vi "柱塞泵调试界面.vi"() -> ()   [LabVIEW 2016, in "质控单元.lvlib"]
uses:
  <vilib>/Utility/miscctls.llb/LVPointTypeDef.ctl
  <vilib>/Analysis/6fits.llb/Curve Fitting Criteria.ctl
  <vilib>/Utility/config.llb/Write Key (U32).vi
  <vilib>/Analysis/NI_AALPro.lvlib
  <vilib>/Utility/config.llb/NI_LVConfig.lvlib
panel:
  out "关闭 2":bool=TRUE
  in  "枚举":enum16{"柱塞泵1", "柱塞泵2", "柱塞泵3", "柱塞泵4"}(ring)
  in  "柱塞泵4":bool
  in  "柱塞泵3":bool
  in  "柱塞泵2":bool
  in  "柱塞泵1":bool
  in  "注出体积选择":u16(ring) items=["0.1mL", "0.3mL", "0.5mL", "0.8mL", "1.0mL"]
  out "线性值":T1
  in  "读取":bool
  in  "写入":bool
  in  "柱塞泵枚举":enum16{"柱塞泵1", "柱塞泵2", "柱塞泵3", "柱塞泵4"}(ring)
  in  "启用计算":bool
  in  "标准体积 2":dbl
  in  "标准体积 3":dbl
  in  "实际体积 1":dbl
  in  "实际体积 2":dbl
  in  "实际体积 3":dbl
  in  "标准体积 4":dbl
  in  "实际体积 4":dbl
  in  "标准体积 5":dbl
  in  "实际体积 5":dbl
  in  "标准体积 1":dbl
  out "拟合方程":string
  out "r^2":dbl format="%_6g"
  in  "B 4":dbl caption="B4"
  in  "K 4":dbl caption="K4"
  in  "B 3":dbl caption="B3"
  in  "K 3":dbl caption="K3"
  in  "B 2":dbl caption="B2"
  in  "K 2":dbl caption="K2"
  in  "B":dbl caption="B1"
  in  "K":dbl caption="K1"
  in  "关闭":bool
  # "柱塞泵手动调试计算界面"
  # "柱塞泵启动控制"
  # "柱塞泵5点线性计算"
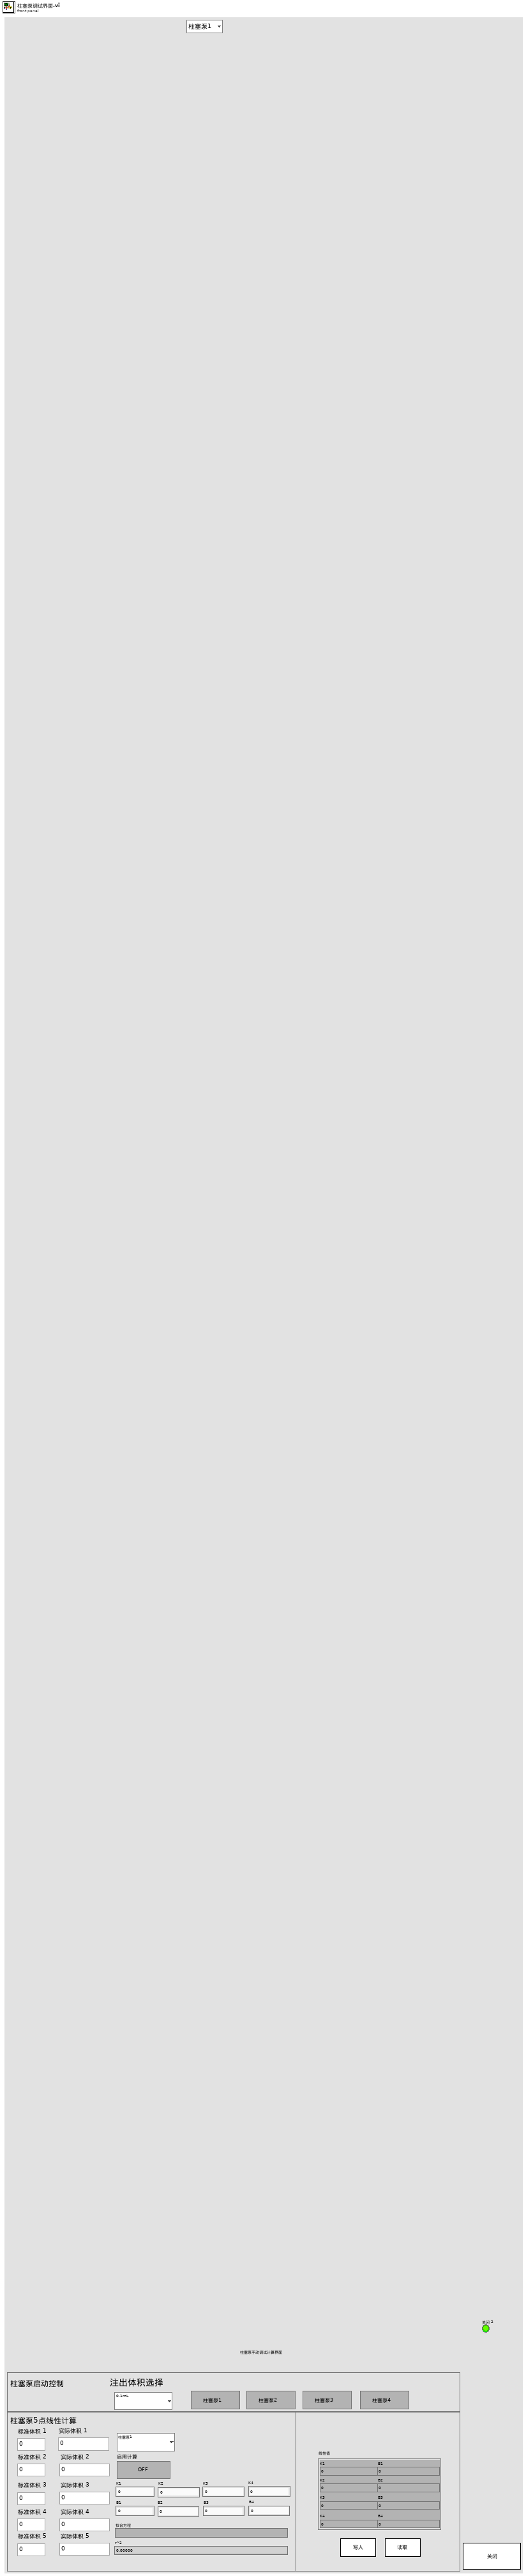
[diagram p1: front panel]
types:
  T1 = cluster{"K1":sgl, "B1":sgl, "K2":sgl, "B2":sgl, "K3":sgl, "B3":sgl, "K4":sgl, "B4":sgl}
  T2 = typedef "LVPointTypeDef.ctl" = cluster{"Horizontal":i16, "Vertical":i16}
  T3 = typedef "NI_LVConfig.lvlib/Config Data RefNum.ctl" = refnum<k1>
  T4 = typedef "NI_AALPro.lvlib/Curve Fitting Criteria.ctl" = u16
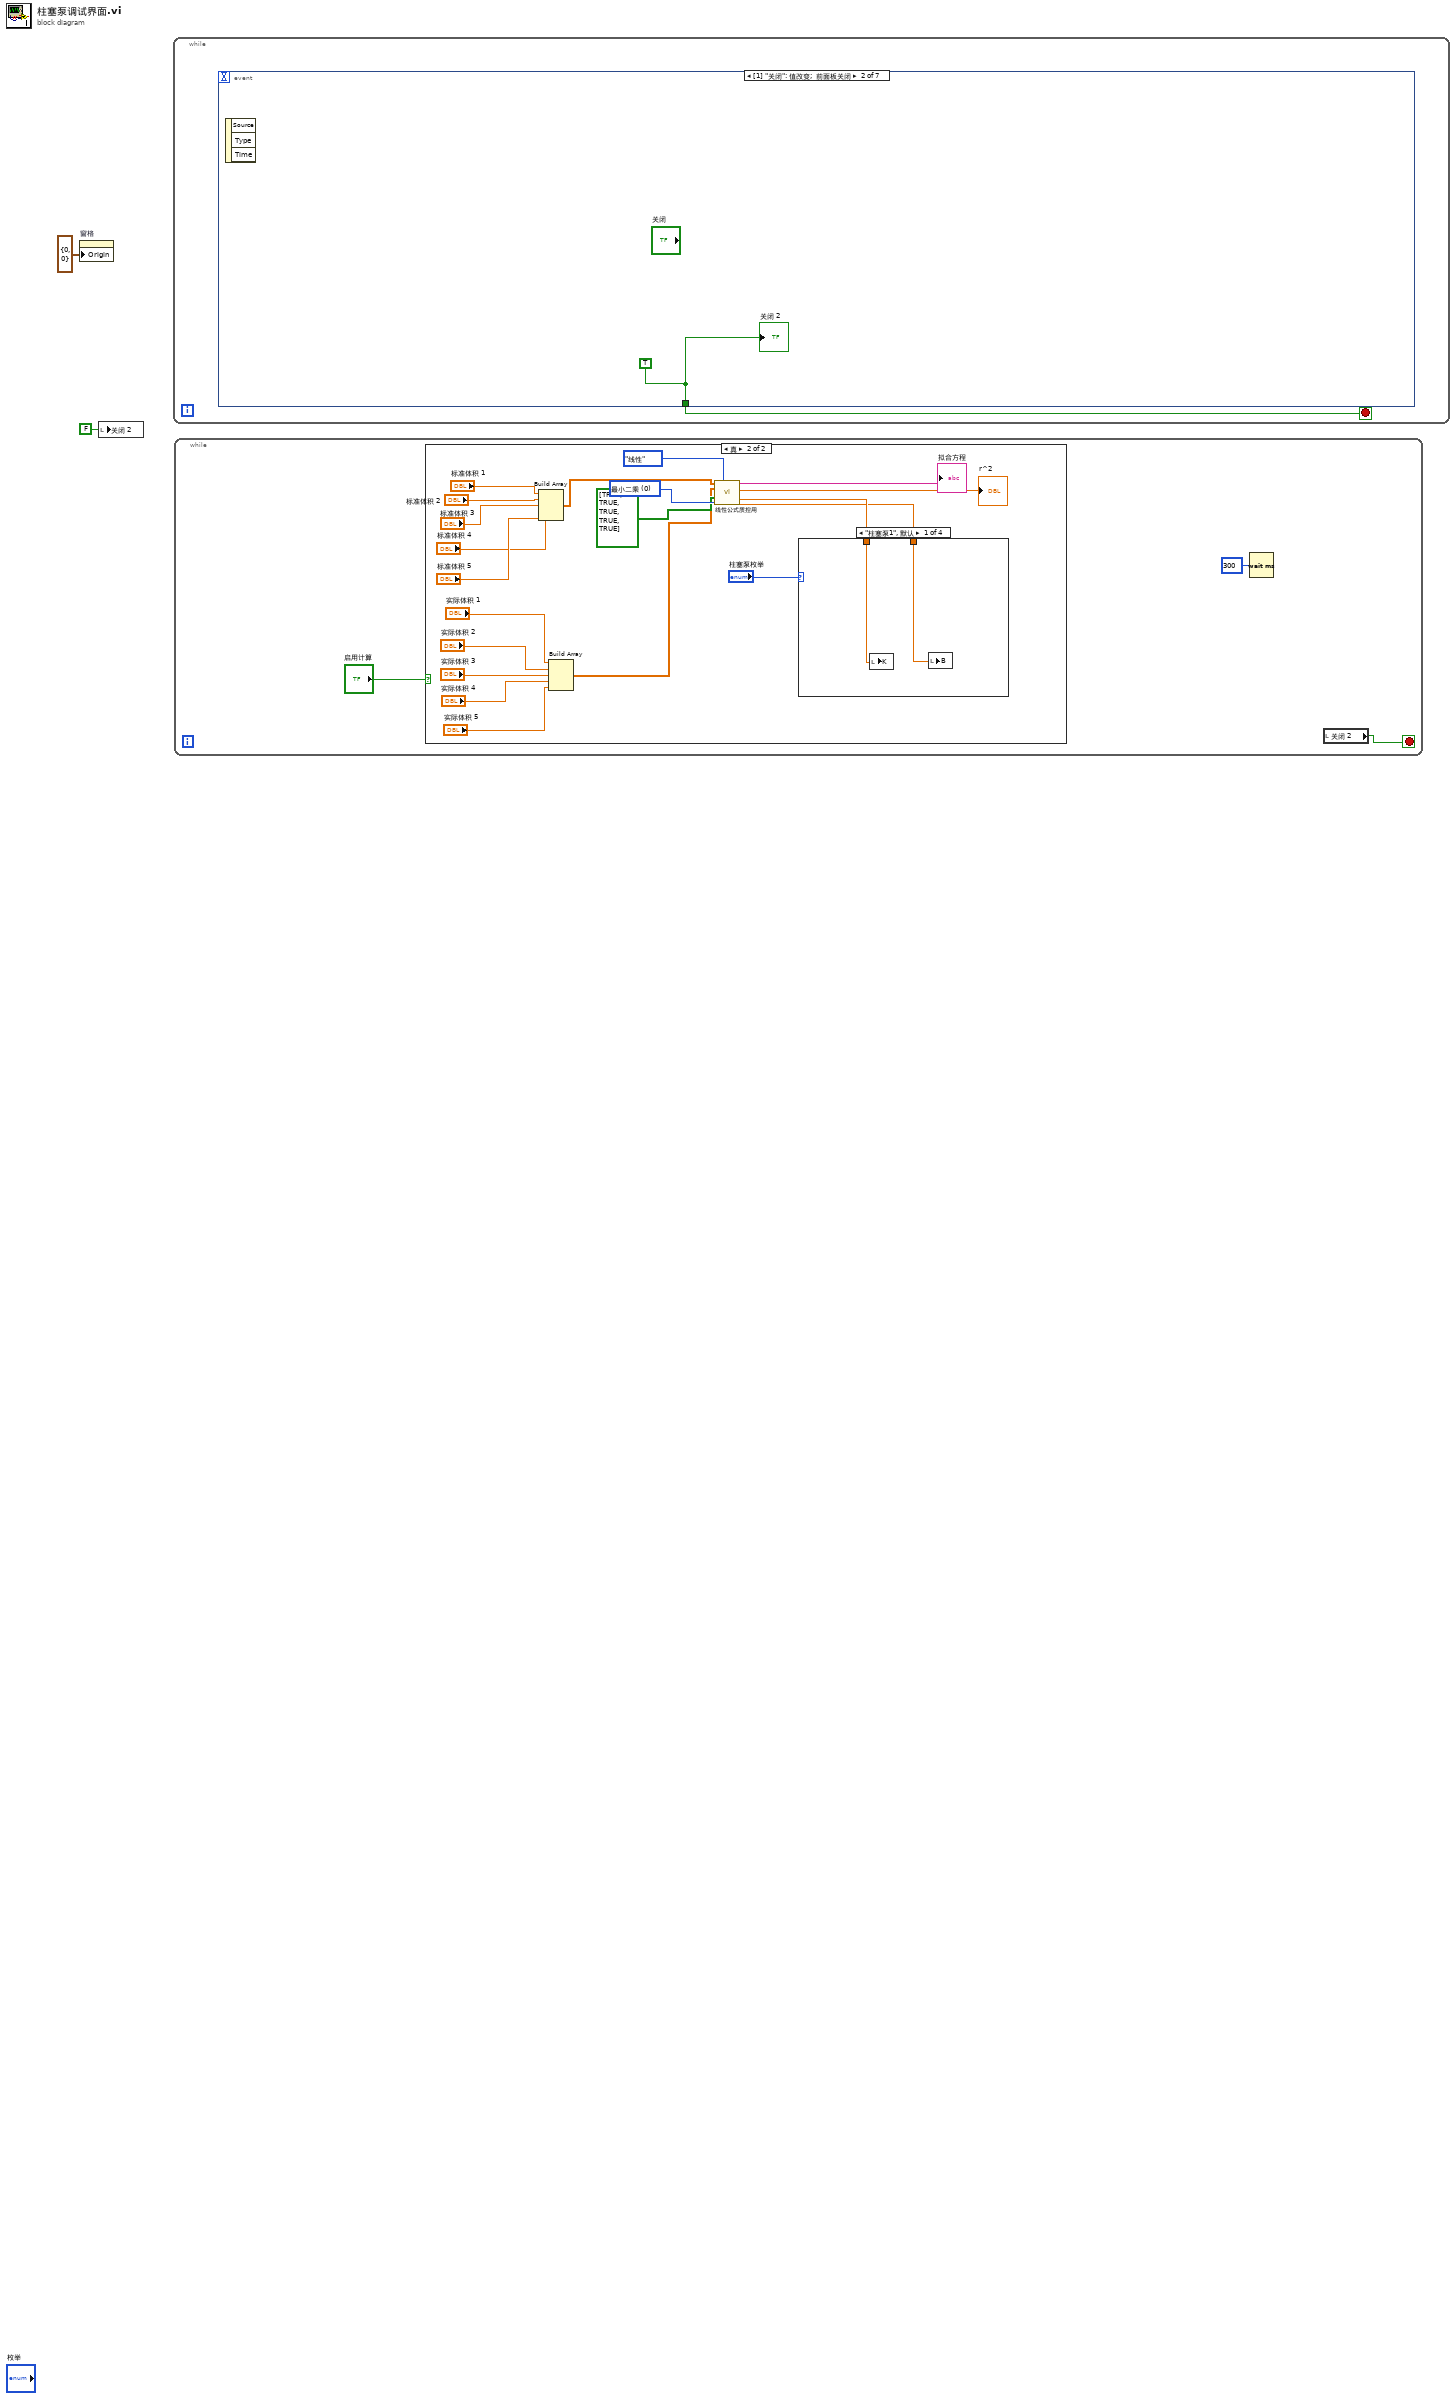
[diagram p0: block diagram]
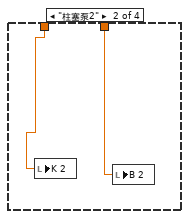
[diagram p3: hidden frame]
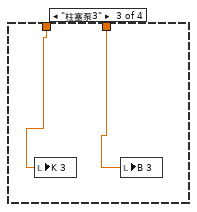
[diagram p4: hidden frame]
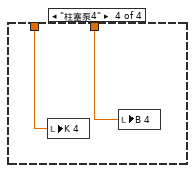
[diagram p5: hidden frame]
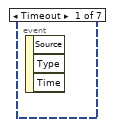
[diagram p6: hidden frame]
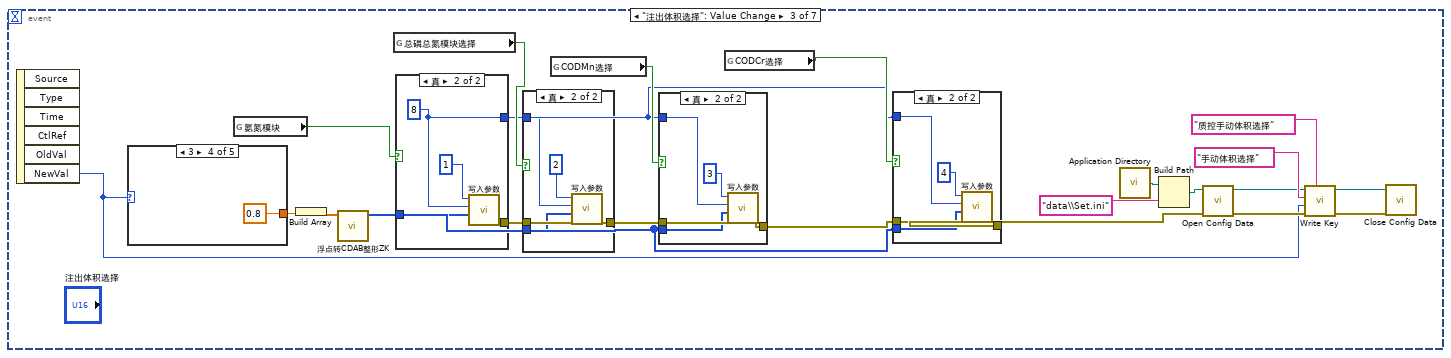
[diagram p7: hidden frame]
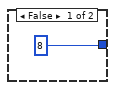
[diagram p9: hidden frame]
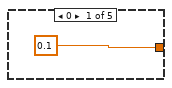
[diagram p12: hidden frame]
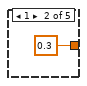
[diagram p13: hidden frame]
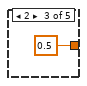
[diagram p14: hidden frame]
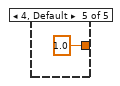
[diagram p15: hidden frame]
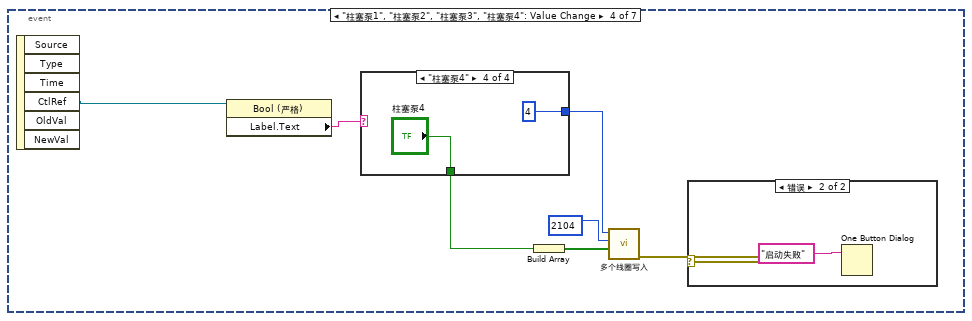
[diagram p16: hidden frame]
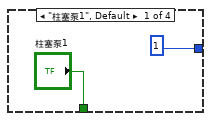
[diagram p17: hidden frame]
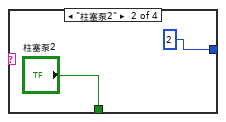
[diagram p18: hidden frame]
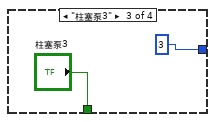
[diagram p19: hidden frame]
diagram:
  n1 = property on="窗格" class="Pane"("Origin"=T2 {"Horizontal"=0, "Vertical"=0} ("原点")) -> ()  [unwired: 2 in, 2 out]
  n2 = local write "关闭 2"(FALSE ("关闭 2")) -> ()
  n3 = while {
    stop <- w3 stop-if-true
    n4 = event shown="[1] \"关闭\": 值改变;  前面板关闭" {
      selector: _ -> [_ _ _ _ _ _ _]
      dyn-events: _ -> [_ _ _ _ _ _ _]
      timeout: _ -> [_ _ _ _ _ _ _]
      tunnel: [_ w4 _ _ _ _ _] -> w3
      event Timeout {
        n5 = event-data() -> ()  [unwired: 1 in, 3 out]
      }
      event "关闭": Value Change; Panel Close {
        w4 = TRUE ("关闭")
        n6 = event-data() -> ()  [unwired: 1 in, 3 out]
        "关闭 2" <- w4
      }
      event "注出体积选择": Value Change {
        n7 = event-data() -> ("NewVal"=w5:u16)  [unwired: 1 in, 5 out]
        n8 = case shown="3" w5 {
          tunnel: [0.1 0.3 0.5 0.8 1.0] -> w8
          frame 0 {
          }
          frame 1 {
          }
          frame 2 {
          }
          frame 3 {
          }
          frame 4, Default {
          }
        }
        n9 = global read "断电保存全局.vi" "氨氮模块"() -> (w23:bool)
        n10 = Build Array(w8) -> (w18:dbl[])
        n11 = call "浮点转CDAB整形ZK.vi"("浮点数"=w18) -> ("CDAB整形输出"=w21:u16[])  [unwired: 10 in]
        n12 = global read "断电保存全局.vi" "总磷总氮模块选择"() -> (w24:bool)
        n13 = case shown="真" w23 {
          tunnel: [_ w36] -> w6
          tunnel: [u16 8 ("starting address") w35] -> w19
          tunnel: w21 -> [_ w34]
          frame False {
          }
          frame True {
            w35 = u16 8 ("starting address")
            n14 = call "写入参数.vi"("values"=w34, "starting address"=w35, "Slave ID"=u8 1) -> ("error out"=w36:errorcluster)  [unwired: 8 in]
          }
        }
        n15 = case shown="真" w24 {
          tunnel: w6 -> [w38 w42]
          tunnel: [w38 w41] -> w7
          tunnel: w19 -> [_ w40]
          tunnel: w21 -> [_ w39]
          frame False {
          }
          frame True {
            n16 = call "写入参数.vi"("Error in"=w42, "values"=w39, "starting address"=w40, "Slave ID"=u8 2) -> ("error out"=w41:errorcluster)  [unwired: 7 in]
          }
        }
        n17 = global read "断电保存全局.vi" "CODMn选择"() -> (w25:bool)
        n18 = case shown="真" w25 {
          tunnel: w7 -> [w44 w48]
          tunnel: w19 -> [_ w47]
          tunnel: [w44 w46] -> w20
          tunnel: w21 -> [_ w45]
          frame False {
          }
          frame True {
            n19 = call "写入参数.vi"("Error in"=w48, "values"=w45, "starting address"=w47, "Slave ID"=u8 3) -> ("error out"=w46:errorcluster)  [unwired: 7 in]
          }
        }
        n20 = global read "断电保存全局.vi" "CODCr选择"() -> (w26:bool)
        n21 = case shown="真" w26 {
          tunnel: w20 -> [w27 w31]
          tunnel: w19 -> [_ w30]
          tunnel: [w27 w29] -> w22
          tunnel: w21 -> [_ w28]
          frame False {
          }
          frame True {
            n22 = call "写入参数.vi"("Error in"=w31, "values"=w28, "starting address"=w30, "Slave ID"=u8 4) -> ("error out"=w29:errorcluster)  [unwired: 7 in]
          }
        }
        n23 = call <vilib>:"Application Directory.vi"() -> ("Application Directory"=w9:path)
        n24 = Build Path(base path=w9, name or relative path="data\\Set.ini" ("名称或相对路径")) -> (appended path=w11:path)
        n25 = call <vilib>:"Open Config Data.vi"("error in (no error)"=w22, "configuration file path"=w11) -> ("error out"=w15:errorcluster, "refnum"=w14:T3)  [unwired: 7 in, 1 out]
        n26 = call-poly <vilib>:"Write Key.vi"("section"="质控手动体积选择", "error in (no error)"=w15, "value"=w5, "key"="手动体积选择" ("section"), "refnum"=w14) -> ("error out"=w13:errorcluster, "refnum out"=w12:T3)  [unwired: 4 in, 1 out]
        n27 = call <vilib>:"Close Config Data.vi"("error in (no error)"=w13, "refnum"=w12) -> ()  [unwired: 8 in, 2 out]
      }
      event "柱塞泵1", "柱塞泵2", "柱塞泵3", "柱塞泵4": Value Change {
        n28 = event-data() -> ("CtlRef"=w56:refnum<vi>)  [unwired: 1 in, 5 out]
        n29 = property class="Bool (严格)"(reference=w56) -> ("Label.Text"=w60:string)  [unwired: 1 in, 2 out]
        n30 = case shown="\"柱塞泵4\"" w60 {
          tunnel: [u8 1 ("Slave ID") u8 2 ("Slave ID") u8 3 ("Slave ID") u8 4 ("Slave ID")] -> w61
          tunnel: ["柱塞泵1" "柱塞泵2" "柱塞泵3" "柱塞泵4"] -> w55
          frame "柱塞泵1", Default {
          }
          frame "柱塞泵2" {
          }
          frame "柱塞泵3" {
          }
          frame "柱塞泵4" {
          }
        }
        n31 = Build Array(w55) -> (w58:bool[])
        n32 = call "多个线圈写入.vi"("values"=w58, "starting address"=u16 2104, "Slave ID"=w61) -> ("error out"=w59:errorcluster)  [unwired: 8 in]
        n33 = case shown="错误" w59 {
          frame No Error {
          }
          frame Error {
            n34 = One Button Dialog(message="启动失败" ("消息")) -> ()  [unwired: 1 in, 1 out]
          }
        }
      }
      event "标准体积 1", "实际体积 5", "标准体积 5", "实际体积 4", "标准体积 4", "实际体积 3", "实际体积 2", "实际体积 1", "标准体积 3", "标准体积 2", "线性值.K1", "线性值.B1", "线性值.K2", "线性值.B2", "线性值.K3", "线性值.B3", "线性值.K4", "线性值.B4": Mouse Down {
        n35 = event-data() -> ("CtlRef"=w74:refnum<vi>)  [unwired: 1 in, 7 out]
        n36 = property class="DigNum"(reference=w74) -> (reference out=w75:refnum<vi>, "Value"=w72:variant)  [unwired: 1 in, 1 out]
        n37 = Variant To Data(type=sgl 0.0 ("NewNumber"), Variant=w72) -> (data=w71:sgl)  [unwired: 1 in, 1 out]
        n38 = call "数字键盘.vi"("OldNumber"=w71) -> ("NewNumber"=w76:sgl)
        n39 = property class="DigNum"(reference=w75, "Val(Sgnl)"=w76) -> ()  [unwired: 1 in, 2 out]
      }
      event "写入": Value Change {
        n40 = event-data() -> ()  [unwired: 1 in, 6 out]
        n41 = control-ref of="柱塞泵枚举"() -> (w80:refnum<vi>)
        n42 = property class="Enum (严格)"(reference=w80) -> ("RingText.Text"=w79:string)  [unwired: 1 in, 2 out]
        n43 = Concatenate Strings("是否将K、B值写入" ("字符串"), w79, "？" ("字符串")) -> (w77:string)
        n44 = Two Button Dialog(message=w77) -> (T button?=w82:bool)  [unwired: 2 in]
        n45 = case shown="真" w82 {
          frame False {
          }
          frame True {
            n46 = local read "柱塞泵枚举"() -> (w83:enum16{"柱塞泵1", "柱塞泵2", "柱塞泵3", "柱塞泵4"})
            n47 = case shown="\"柱塞泵4\"" w83 {
              tunnel: [w88 w99 w109 w119] -> w84
              frame "柱塞泵1", Default {
                w85 = 0 ("索引")
                n48 = Build Array("K", "B") -> (w91:dbl[])
                n49 = call "浮点转CDAB整形ZK.vi"("浮点数"=w91) -> ("CDAB整形输出"=w93:u16[])  [unwired: 10 in]
                n50 = Build Array(w85) -> (w92:i32[])
                n51 = Insert Into Array(array=w92, index=w85, new element=w93) -> (w94:i32[])
                n52 = call "写入参数.vi"("values"=w94, "starting address"=u16 1, "Slave ID"=u8 1) -> ("error out"=w88:errorcluster)  [unwired: 8 in]
              }
              frame "柱塞泵2" {
                w97 = 0 ("索引")
                n53 = Build Array("K 2", "B 2") -> (w102:dbl[])
                n54 = Build Array(w97) -> (w100:i32[])
                n55 = call "浮点转CDAB整形ZK.vi"("浮点数"=w102) -> ("CDAB整形输出"=w103:u16[])  [unwired: 10 in]
                n56 = Insert Into Array(array=w100, index=w97, new element=w103) -> (w104:i32[])
                n57 = call "写入参数.vi"("values"=w104, "starting address"=u16 1, "Slave ID"=u8 2) -> ("error out"=w99:errorcluster)  [unwired: 8 in]
              }
              frame "柱塞泵3" {
                w107 = 0 ("索引")
                n58 = Build Array("K 3", "B 3") -> (w113:dbl[])
                n59 = Build Array(w107) -> (w112:i32[])
                n60 = call "浮点转CDAB整形ZK.vi"("浮点数"=w113) -> ("CDAB整形输出"=w114:u16[])  [unwired: 10 in]
                n61 = Insert Into Array(array=w112, index=w107, new element=w114) -> (w111:i32[])
                n62 = call "写入参数.vi"("values"=w111, "starting address"=u16 1, "Slave ID"=u8 3) -> ("error out"=w109:errorcluster)  [unwired: 8 in]
              }
              frame "柱塞泵4" {
                n63 = Build Array(0 ("背隙补偿步数")) -> (w122:i32[])
                n64 = Build Array("K 4", "B 4") -> (w124:dbl[])
                n65 = call "浮点转CDAB整形ZK.vi"("浮点数"=w124) -> ("CDAB整形输出"=w125:u16[])  [unwired: 10 in]
                n66 = Insert Into Array(array=w122, index=0 ("索引"), new element=w125) -> (w121:i32[])
                n67 = call "写入参数.vi"("values"=w121, "starting address"=u16 1, "Slave ID"=u8 4) -> ("error out"=w119:errorcluster)  [unwired: 8 in]
              }
            }
            n68 = case shown="无错误" w84 {
              frame No Error {
                n69 = One Button Dialog(message="写入成功" ("消息"), button name ("OK")="确定" ("按钮名称（“确定”）")) -> ()  [unwired: 1 out]
              }
              frame Error {
                n70 = One Button Dialog(message="写入失败" ("消息"), button name ("OK")="确定" ("按钮名称（“确定”）")) -> ()  [unwired: 1 out]
              }
            }
          }
        }
      }
      event "读取": Value Change {
        n71 = event-data() -> ()  [unwired: 1 in, 6 out]
        n72 = local read "线性值"() -> (w148:T1)
        n73 = global read "断电保存全局.vi" "氨氮模块"() -> (w146:bool)
        n74 = case shown="假" w146 {
          tunnel: [errorcluster {"status"=FALSE, "code"=0, "source"=""} ("error out") w170] -> w130
          tunnel: [w164 w167] -> w132
          tunnel: [w163 w166] -> w133
          tunnel: w148 -> [w162 _]
          frame False {
            n75 = Unbundle By Name(w162) -> ("K1"=w164:sgl, "B1"=w163:sgl)
          }
          frame True {
            n76 = call "读取参数.vi"("Slave ID"=u8 1, "starting address"=u16 1, "quantity"=u16 4) -> ("values"=w169:u16[], "error out"=w170:errorcluster)  [unwired: 6 in]
            n77 = call "浮点CDAB转换质控.vi"("数组"=w169) -> ("数组 2"=w168:sgl[])  [unwired: 10 in]
            n78 = Index Array(array=w168) -> (element #1=w167:sgl, element #2=w166:sgl)  [unwired: 2 in]
          }
        }
        n79 = global read "断电保存全局.vi" "总磷总氮模块选择"() -> (w145:bool)
        n80 = case shown="假" w145 {
          tunnel: w130 -> [w175 w185]
          tunnel: [w175 w184] -> w131
          tunnel: [w177 w181] -> w134
          tunnel: [w176 w180] -> w135
          tunnel: w148 -> [w174 _]
          frame False {
            n81 = Unbundle By Name(w174) -> ("K2"=w177:sgl, "B2"=w176:sgl)
          }
          frame True {
            n82 = call "读取参数.vi"("Slave ID"=u8 2, "starting address"=u16 1, "quantity"=u16 4, "Error in"=w185) -> ("values"=w183:u16[], "error out"=w184:errorcluster)  [unwired: 5 in]
            n83 = call "浮点CDAB转换质控.vi"("数组"=w183) -> ("数组 2"=w182:sgl[])  [unwired: 10 in]
            n84 = Index Array(array=w182) -> (element #1=w181:sgl, element #2=w180:sgl)  [unwired: 2 in]
          }
        }
        n85 = global read "断电保存全局.vi" "CODMn选择"() -> (w144:bool)
        n86 = case shown="假" w144 {
          tunnel: w131 -> [w188 w198]
          tunnel: [w190 w195] -> w136
          tunnel: [w189 w194] -> w137
          tunnel: [w188 w191] -> w139
          tunnel: w148 -> [w187 _]
          frame False {
            n87 = Unbundle By Name(w187) -> ("K3"=w190:sgl, "B3"=w189:sgl)
          }
          frame True {
            n88 = call "读取参数.vi"("Slave ID"=u8 3, "starting address"=u16 1, "quantity"=u16 4, "Error in"=w198) -> ("values"=w197:u16[], "error out"=w191:errorcluster)  [unwired: 5 in]
            n89 = call "浮点CDAB转换质控.vi"("数组"=w197) -> ("数组 2"=w196:sgl[])  [unwired: 10 in]
            n90 = Index Array(array=w196) -> (element #1=w195:sgl, element #2=w194:sgl)  [unwired: 2 in]
          }
        }
        n91 = global read "断电保存全局.vi" "CODCr选择"() -> (w143:bool)
        n92 = case shown="假" w143 {
          tunnel: w139 -> [w150 w160]
          tunnel: [w152 w157] -> w141
          tunnel: [w151 w156] -> w142
          tunnel: [w150 w153] -> w140
          tunnel: w148 -> [w149 _]
          frame False {
            n93 = Unbundle By Name(w149) -> ("K4"=w152:sgl, "B4"=w151:sgl)
          }
          frame True {
            n94 = call "读取参数.vi"("Slave ID"=u8 4, "starting address"=u16 1, "quantity"=u16 4, "Error in"=w160) -> ("values"=w159:u16[], "error out"=w153:errorcluster)  [unwired: 5 in]
            n95 = call "浮点CDAB转换质控.vi"("数组"=w159) -> ("数组 2"=w158:sgl[])  [unwired: 10 in]
            n96 = Index Array(array=w158) -> (element #1=w157:sgl, element #2=w156:sgl)  [unwired: 2 in]
          }
        }
        n97 = Bundle By Name(cluster=T1 {"K1"=0.0, "B1"=0.0, "K2"=0.0, "B2"=0.0, "K3"=0.0, "B3"=0.0, "K4"=0.0, "B4"=0.0} ("线性值"), "K1"=w132, "B1"=w133, "K2"=w134, "B2"=w135, "K3"=w136, "B3"=w137, "K4"=w141, "B4"=w142) -> (→"线性值":T1)
        n98 = case shown="无错误" w140 {
          frame No Error {
            n99 = One Button Dialog(message="读取成功" ("消息"), button name ("OK")="确定" ("按钮名称（“确定”）")) -> ()  [unwired: 1 out]
          }
          frame Error {
            n100 = One Button Dialog(message="读取失败" ("消息"), button name ("OK")="确定" ("按钮名称（“确定”）")) -> ()  [unwired: 1 out]
          }
        }
      }
    }
  }
  n101 = while {
    stop <- w205 stop-if-true
    n102 = case shown="真" "启用计算" {
      frame False {
      }
      frame True {
        w223 = T4 0 items=["最小二乘", "最小绝对残差", "Bisquare"] ("method")
        n103 = Build Array("标准体积 1", "标准体积 2", "标准体积 3", "标准体积 4", "标准体积 5") -> (w220:dbl[])
        n104 = Build Array("实际体积 1", "实际体积 2", "实际体积 3", "实际体积 4", "实际体积 5") -> (w221:dbl[])
        n105 = call "线性公式质控用.vi"("标液浓度"=w220, "模型"=enum32{"线性", "多项式"}."线性", "监测浓度"=w221, "启用"=bool[] [TRUE, TRUE, TRUE, TRUE, TRUE], "method"=w223) -> ("拟合方程"=→"拟合方程":string, "r^2"=→"r^2":dbl, "slope"=w209:dbl, "intercept"=w208:dbl)  [unwired: 6 in, 1 out]
        n106 = case shown="\"柱塞泵1\", 默认" "柱塞泵枚举" {
          tunnel: w209 -> [w227 w230 w231 w234]
          tunnel: w208 -> [w228 w229 w232 w233]
          frame "柱塞泵1", Default {
            n107 = local write "K"(w227) -> ()
            n108 = local write "B"(w228) -> ()
          }
          frame "柱塞泵2" {
            n109 = local write "K 2"(w230) -> ()
            n110 = local write "B 2"(w229) -> ()
          }
          frame "柱塞泵3" {
            n111 = local write "K 3"(w231) -> ()
            n112 = local write "B 3"(w232) -> ()
          }
          frame "柱塞泵4" {
            n113 = local write "K 4"(w234) -> ()
            n114 = local write "B 4"(w233) -> ()
          }
        }
      }
    }
    n115 = Wait (ms)(milliseconds to wait=u32 300 ("等待时间（毫秒）")) -> ()  [unwired: 1 out]
    n116 = local read "关闭 2"() -> (w205:bool)
  }
